vi "Hidden Numbers Integrator.vi"(1 "Integrand":fxp<+/-,18,1> format="%.18g", 2 "Size of Integrator":fxp<+,6,6>) -> (0 "18b (s-fxp-1) out":fxp<+/-,18,1> format="%.18g")   [LabVIEW 2010]
panel:
  out "64b (s-fxp-47) Post Addition":fxp<+/-,64,47> format="%.32g"
  out "64b (s-fxp-47) Next Time":fxp<+/-,64,47> format="%.32g"
  out "64b (s-fxp-47) Internal":fxp<+/-,64,47> format="%.32g"
  # "64b (s-fxp-47) internal representation"
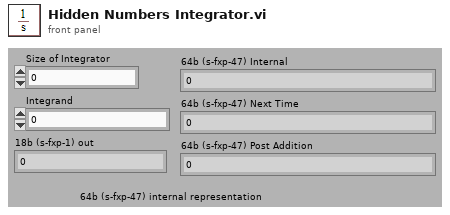
[diagram p1: front panel]
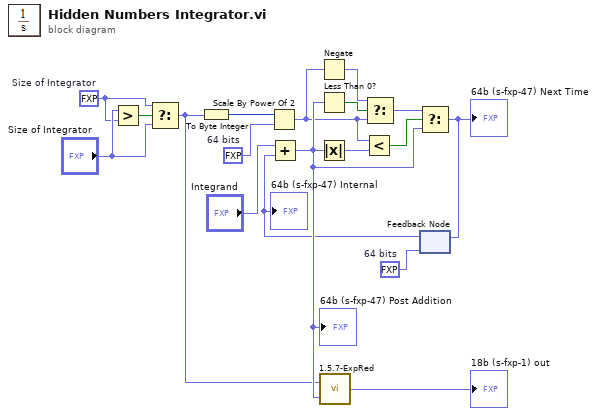
[diagram p0: block diagram]
diagram:
  w1 = fxp<+,6,6> 45.0  # Size of Integrator
  w8 = fxp<+/-,64,47> 1.0  # 64 bits
  w5 = fxp<+/-,64,47> 0.0  # 64 bits
  n1 = Greater?(x="Size of Integrator", y=w1) -> (0:w2:bool)
  n2 = Select(t=w1, s=w2, f="Size of Integrator") -> (s? t:f=w3:fxp<+,6,6>)
  n3 = To Byte Integer(number=w3) -> (8bit integer=w17:i8)
  n4 = Scale By Power Of 2(n=w17, x=w8) -> (x*2^n=w13:fxp<+/-,64,47>)
  n5 = Negate(x=w13) -> (-x=w12:fxp<+/-,64,47>)
  n6 = feedback #1(w5) -> (w6:fxp<+/-,64,47>)
  "64b (s-fxp-47) Internal" <- w6
  n7 = Add(x="Integrand", y=w6) -> (x+y=w16:fxp<+/-,64,47>)
  "64b (s-fxp-47) Post Addition" <- w16
  n8 = Less Than 0?(x=w16) -> (x < 0?=w11:bool)
  n9 = Absolute Value(x=w16) -> (abs(x)=w9:fxp<+,64,47>)
  n10 = call "1.5.7-ExpRed.vi"("64b (s-fxp-47) in"=w16, "N"=w3) -> ("18b (s-fxp-1) out"=→"18b (s-fxp-1) out":fxp<+/-,18,1>)
  n11 = Less?(x=w13, y=w9) -> (x < y?=w10:bool)
  n12 = Select(t=w12, s=w11, f=w13) -> (s? t:f=w14:fxp<+/-,64,47>)
  n13 = Select(t=w14, s=w10, f=w16) -> (s? t:f=w15:fxp<+/-,64,47>)
  "64b (s-fxp-47) Next Time" <- w15
  n14 = feedback-in #1(w15) -> ()
